vi "Equate Actor Inputs.vi"(9 "Actor":refnum<class "Actor.lvclass">, 10 "Actor":refnum<class "Actor.lvclass">) -> (2 "Equal":bool)   [LabVIEW 2020, in "jettl.lvlib"]
uses:
  jettl.lvlib
  Actor/Actor.lvclass
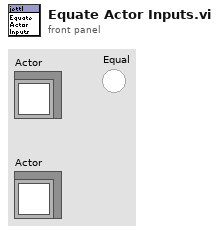
[diagram p1: front panel]
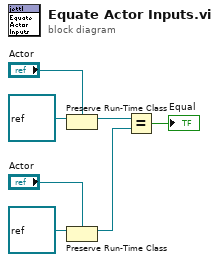
[diagram p0: block diagram]
diagram:
  n1 = Preserve Run-Time Class(object in=refnum<class> refnum ("LabVIEW Object"), 2:"Actor") -> (object out=w3:refnum<class "Actor.lvclass">)  [unwired: 1 in, 1 out]
  n2 = Preserve Run-Time Class(object in=refnum<class> refnum ("LabVIEW Object"), 2:"Actor") -> (object out=w2:refnum<class "Actor.lvclass">)  [unwired: 1 in, 1 out]
  n3 = Equal?(x=w3, y=w2) -> (x = y?=→"Equal":bool)
